vi "pARSADFASF.vi"(11 "String in 3":string="${case${select}.addr}+${protocol}://${ip}:${port}") -> (3 "Array":string[](array[string]))   [LabVIEW 2017]
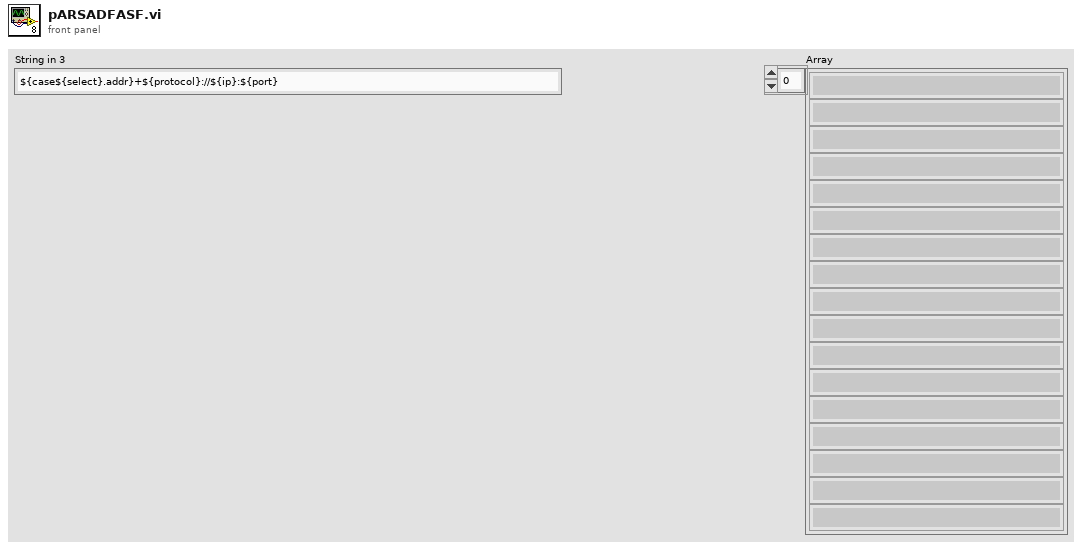
[diagram p1: front panel]
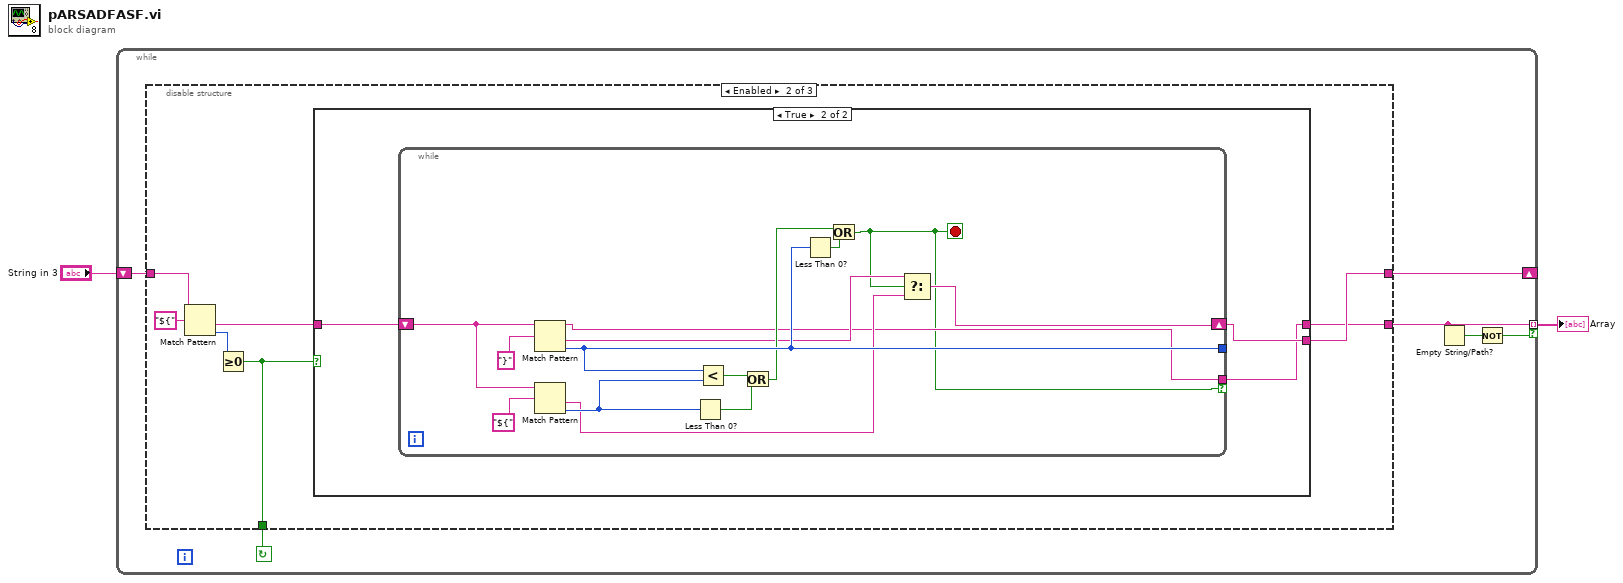
[diagram p0: block diagram]
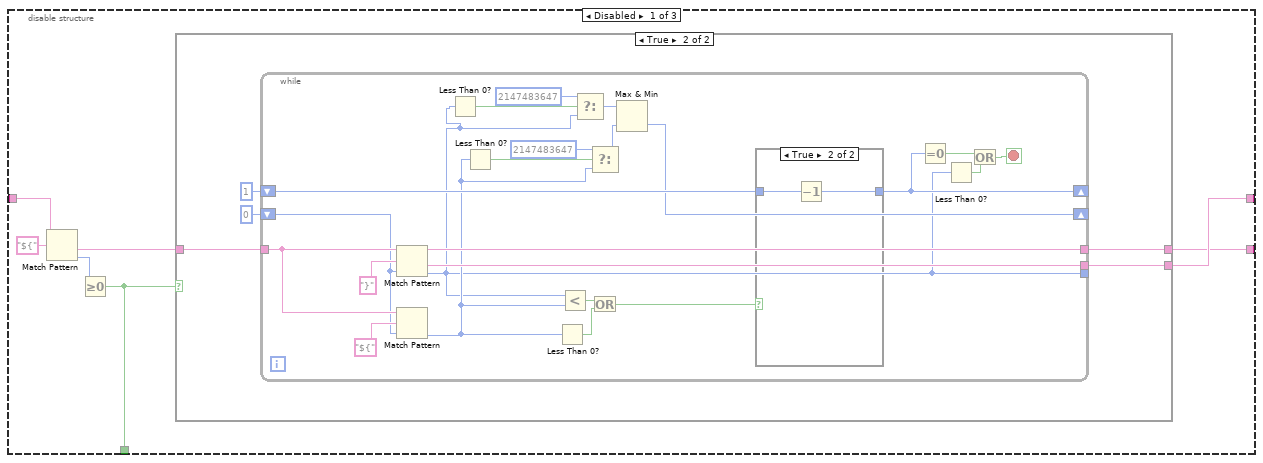
[diagram p2: hidden frame]
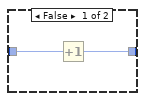
[diagram p4: hidden frame]
diagram:
  n1 = while {
    shift-right: [w7] -> _
    shift-left: "String in 3" -> [w8]
    tunnel: [w4] -> w1 mode=indexing if=w3
    stop <- w6 continue-if-true
    n2 = disable-structure shown="Enabled" {
      disable-tunnel: w8 -> [w13 w50 _]
      disable-tunnel: [w12 w54 _] -> w7
      disable-tunnel: [w10 w52 _] -> w6
      disable-tunnel: [w9 w51 _] -> w4
      frame Disabled {
        n3 = Match Pattern(string=w13, regular expression="${") -> (after substring=w14:string, offset past match=w11:i32)  [unwired: 1 in, 2 out]
        n4 = Greater Or Equal To 0?(x=w11) -> (x >= 0?=w10:bool)
        n5 = case shown="True" w10 {
          tunnel: w14 -> [w16 w20]
          tunnel: [w16 w21] -> w12
          tunnel: [_ w19] -> w9
          frame False {
          }
          frame True {
            n6 = while {
              tunnel: [w44] -> w21
              tunnel: [w22] -> _
              shift-right: [w31] -> _
              shift-left: 0 ("offset (0)") -> [w40]
              shift-right: [w35] -> _
              shift-left: 1 ("offset (0)") -> [w37]
              tunnel: w20 -> [w41]
              tunnel: [w30] -> w19
              stop <- w34 stop-if-true
              n7 = Match Pattern(string=w41, regular expression="}", offset (0)=w40) -> (before substring=w30:string, after substring=w44:string, offset past match=w22:i32)  [unwired: 1 out]
              n8 = Match Pattern(string=w41, regular expression="${", offset (0)=w40) -> (offset past match=w28:i32)  [unwired: 3 out]
              n9 = Less Than 0?(x=w22) -> (x < 0?=w24:bool)
              n10 = Less Than 0?(x=w28) -> (x < 0?=w29:bool)
              n11 = Less Than 0?(x=w28) -> (x < 0?=w38:bool)
              n12 = Less?(x=w22, y=w28) -> (x < y?=w39:bool)
              n13 = Select(t=2147483647, s=w24, f=w22) -> (s? t:f=w23:i32)
              n14 = Select(t=2147483647, s=w29, f=w28) -> (s? t:f=w26:i32)
              n15 = Or(x=w39, y=w38) -> (x .or. y?=w36:bool)
              n16 = Max & Min(x=w23, y=w26) -> (min(x,y)=w31:i32)  [unwired: 1 out]
              n17 = case shown="True" w36 {
                tunnel: w37 -> [w46 w48]
                tunnel: [w45 w47] -> w35
                frame False {
                  n18 = Increment(x=w46) -> (x+1=w45:i32)
                }
                frame True {
                  n19 = Decrement(x=w48) -> (x-1=w47:i32)
                }
              }
              n20 = Equal To 0?(x=w35) -> (x = 0?=w33:bool)
              n21 = Less Than 0?(x=w22) -> (x < 0?=w32:bool)
              n22 = Or(x=w33, y=w32) -> (x .or. y?=w34:bool)
            }
          }
        }
      }
      frame Enabled {
        n23 = Match Pattern(string=w50, regular expression="${") -> (after substring=w49:string, offset past match=w53:i32)  [unwired: 1 in, 2 out]
        n24 = Greater Or Equal To 0?(x=w53) -> (x >= 0?=w52:bool)
        n25 = case shown="True" w52 {
          tunnel: w49 -> [w56 w59]
          tunnel: [w56 w58] -> w54
          tunnel: [_ w57] -> w51
          frame False {
          }
          frame True {
            n26 = while {
              tunnel: [w67] -> _
              shift-right: [w62] -> w58
              shift-left: w59 -> [w71]
              tunnel: [w61] -> w57 if=w60
              stop <- w60 stop-if-true
              n27 = Match Pattern(string=w71, regular expression="}") -> (before substring=w61:string, after substring=w63:string, offset past match=w67:i32)  [unwired: 1 in, 1 out]
              n28 = Match Pattern(string=w71, regular expression="${") -> (after substring=w64:string, offset past match=w68:i32)  [unwired: 1 in, 2 out]
              n29 = Less Than 0?(x=w68) -> (x < 0?=w65:bool)
              n30 = Less?(x=w67, y=w68) -> (x < y?=w70:bool)
              n31 = Or(x=w70, y=w65) -> (x .or. y?=w66:bool)
              n32 = Less Than 0?(x=w67) -> (x < 0?=w69:bool)
              n33 = Or(x=w66, y=w69) -> (x .or. y?=w60:bool)
              n34 = Select(t=w63, s=w60, f=w64) -> (s? t:f=w62:string)
            }
          }
        }
      }
      frame Disabled {
      }
    }
    n35 = Empty String/Path?(string/path=w4) -> (empty?=w5:bool)
    n36 = Not(x=w5) -> (.not. x?=w3:bool)
  }
  "Array" <- w1
